vi "Insight_Response_Parser.vi"(8 "error in (no error)":errorcluster, 9 "Command String":string=":CONF:MEASure:WINDow", 11 "Laser Response In":string=":CONF:MEASure:WINDow") -> (0 "error out":errorcluster, 2 "Value":dbl format="%.4g", 3 "Laser Response Out":string=":CONF:MEASure:WINDow")   [LabVIEW 2015]
doc: "Insight Photonic Solutions\n\nThis VI takes in a query response from the Insight laser, and parses it into a numerical value. This subVI only works for returns of a single numerical value. Also, this parser presently handles responses from Atlas 3.1 or earlier, and version 3.2 and later.\n\nINPUTS\nCommand String - this is the exact full SCPI command (without the question mark, if a query) sent to the laser\nLaser Response In - the string response from the laser.\n\nOUTPUTS\nLaser Response Out - this is a pass-through of the Laser Response In\nValue - the parsed value from the response string. This is returned as a Double, but in fact the numerical type may be signed integer, unsigned integer, double, etc. I chose a single type to make the code more universal, but I leave it to the user to correctly typecast the number upon receipt.\n\nver 1.0 - original release"
uses:
  <vilib>/Utility/error.llb/DialogType.ctl
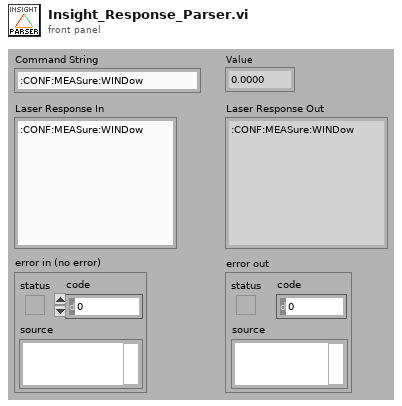
[diagram p1: front panel]
types:
  T1 = typedef "DialogType.ctl" = u16
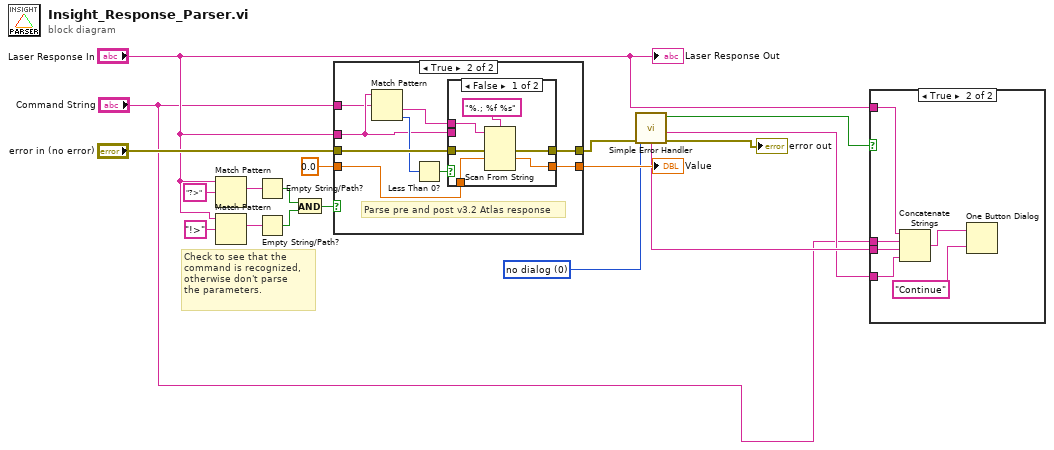
[diagram p0: block diagram]
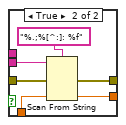
[diagram p4: hidden frame]
diagram:
  w4 = T1 0 items=["no dialog", "OK message", "continue or stop message", "OK message + warnings", "continue/stop + warnings"] ("type of dialog (OK msg:1)")
  # "Check to see that the \ncommand is recognized,\notherwise don't parse \nthe parameters."
  n1 = Match Pattern(string="Laser Response In", regular expression="?>") -> (match substring=w14:string)  [unwired: 1 in, 3 out]
  n2 = Match Pattern(string="Laser Response In", regular expression="!>") -> (match substring=w15:string)  [unwired: 1 in, 3 out]
  n3 = Empty String/Path?(string/path=w14) -> (empty?=w17:bool)
  n4 = Empty String/Path?(string/path=w15) -> (empty?=w18:bool)
  n5 = And(x=w17, y=w18) -> (x .and. y?=w12:bool)
  n6 = case shown="True" w12 {
    tunnel: [w20 w27] -> w8
    tunnel: "error in (no error)" -> [w20 w26]
    tunnel: "Laser Response In" -> [_ w23]
    tunnel: [w19 w28] -> w9
    tunnel: "Command String" -> [_ w22]
    tunnel: 0.0 ("default value 1") -> [w19 w21]
    frame False {
    }
    frame True {
      # "Parse pre and post v3.2 Atlas response"
      n7 = Match Pattern(string=w23, regular expression=w22) -> (after substring=w24:string, offset past match=w25:i32)  [unwired: 1 in, 2 out]
      n8 = Less Than 0?(x=w25) -> (x < 0?=w29:bool)
      n9 = case shown="False" w29 {
        tunnel: w24 -> [w34 _]
        tunnel: w23 -> [_ w40]
        tunnel: [w35 w41] -> w27
        tunnel: [w32 w38] -> w28
        tunnel: w26 -> [w31 w37]
        tunnel: w21 -> [w30 w36]
        frame False {
          n10 = Scan From String(format string="%.; %f %s" ("f"), input string=w34, error in=w31, default 1=w30) -> (error out=w35:errorcluster, output 1=w32:dbl)  [unwired: 3 in, 2 out]
        }
        frame True {
          n11 = Scan From String(format string="%.;%[^:]: %f", input string=w40, error in=w37, default 2=w36) -> (error out=w41:errorcluster, output 2=w38:dbl)  [unwired: 3 in, 2 out]
        }
      }
    }
  }
  "Value" <- w9
  n12 = call <vilib>:"Simple Error Handler.vi"("type of dialog (OK msg:1)"=w4, "error in (no error)"=w8) -> ("error?"=w6:bool, "source out"=w2:string, "error out"=→"error out":errorcluster, "message"=w3:string)  [unwired: 3 in, 1 out]
  n13 = case shown="True" w6 {
    tunnel: "Laser Response In" -> [_ w47]
    tunnel: "Command String" -> [_ w46]
    tunnel: w3 -> [_ w44]
    tunnel: w2 -> [_ w43]
    frame False {
    }
    frame True {
      n14 = Concatenate Strings(w47, w46, w44, w43) -> (w45:string)
      n15 = One Button Dialog(message=w45, button name ("OK")="Continue") -> ()  [unwired: 1 out]
    }
  }
  "Laser Response Out" <- "Laser Response In"
